vi "VIP_Post-Install Custom Action 2021.vi"(10 "Variant":variant) -> (0 "error out":errorcluster)   [LabVIEW 2021]
uses:
  <vilib>/Utility/sysdir.llb/System Directory Type.ctl
  <userlib>/_OpenG.lib/file/file.llb/Build Path - Traditional__ogtk.vi
  <userlib>/_OpenG.lib/lvzip/fileutil.llb/subVIs/FILE Rename (Path)__ogtk.vi
  <userlib>/_OpenG.lib/file/file.llb/File Exists - Scalar__ogtk.vi
  <resource>/dialog/lvconfig.llb/LV Config Read String.vi
  <resource>/dialog/lvconfig.llb/LV Config Write String.vi
  <vilib>/regexp/Match Regular Expression.xnode
  <userlib>/_OpenG.lib/file/file.llb/openg_file.lvlib
panel:
  # "POST INSTALL"
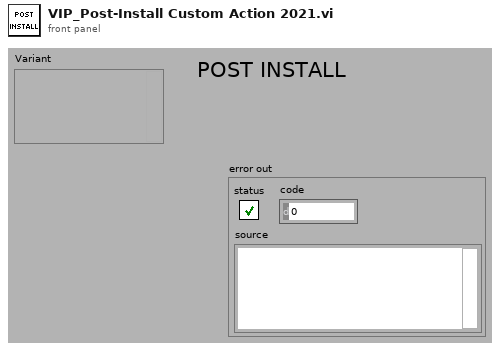
[diagram p1: front panel]
types:
  T1 = enum16{"open", "replace", "create", "open or create", "replace or create", "replace or create with confirmation"}
  T2 = typedef "System Directory Type.ctl" = i32
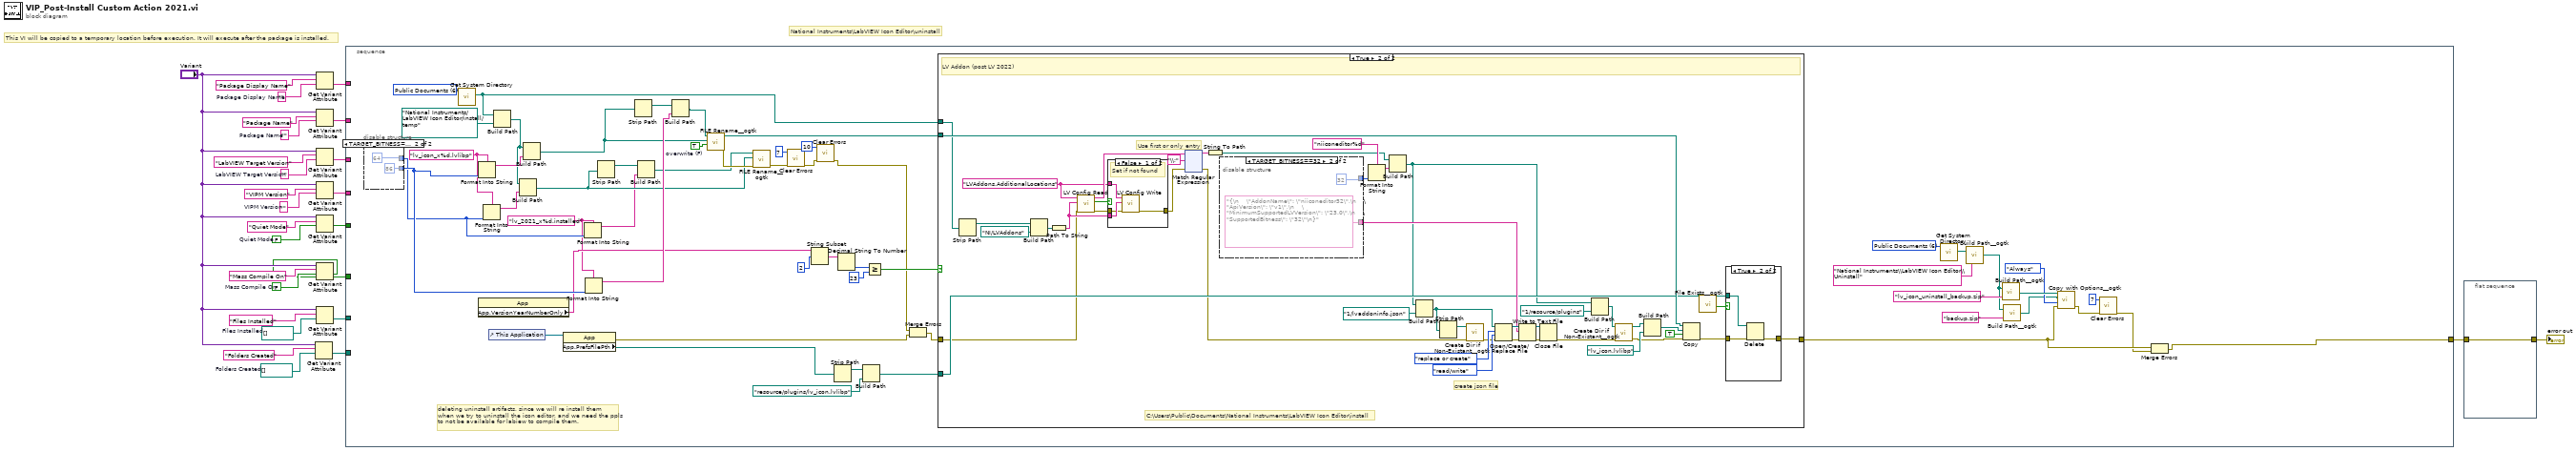
[diagram p0: block diagram]
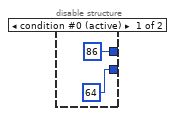
[diagram p2: hidden frame]
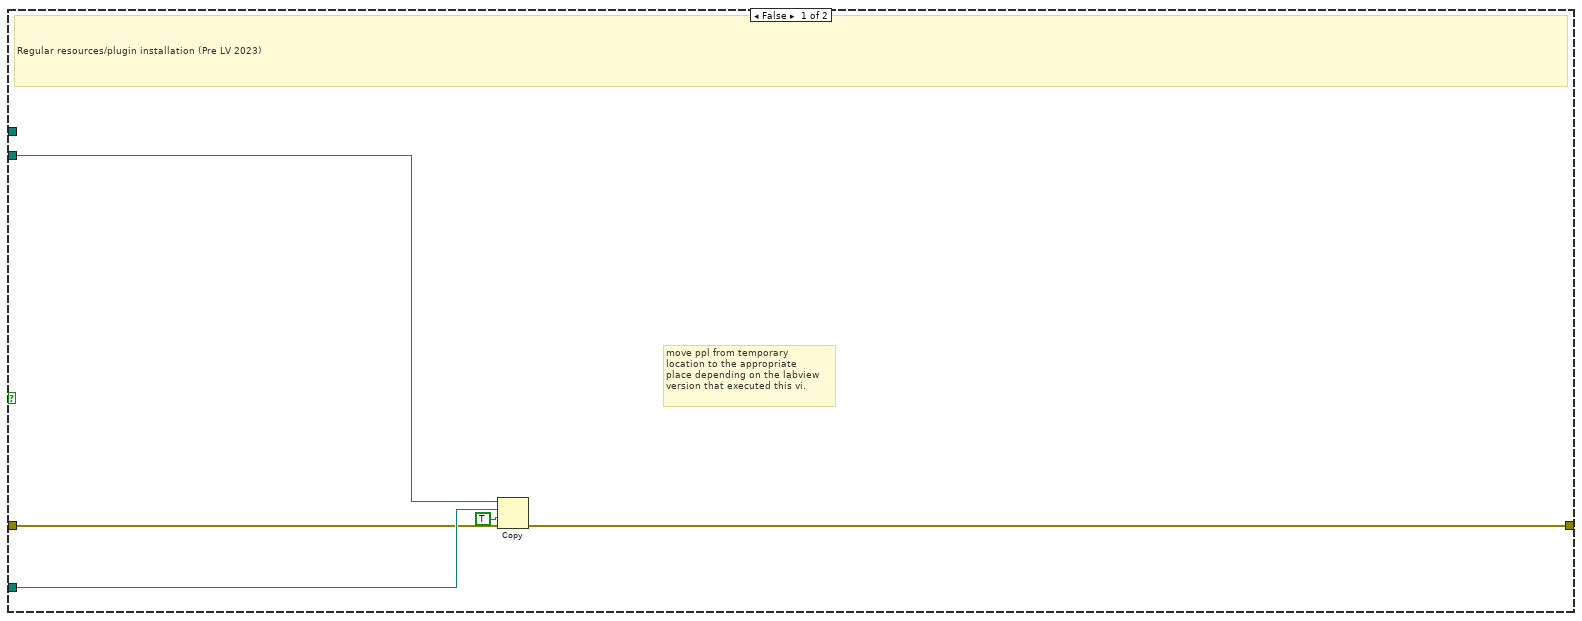
[diagram p3: hidden frame]
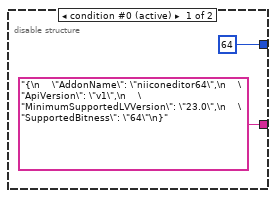
[diagram p6: hidden frame]
diagram:
  w11 = path[] []  # Folders Created
  w12 = path[] []  # Files Installed
  w16 = FALSE  # Mass Compile On
  w17 = ""  # Package Display Name
  w18 = FALSE  # Quiet Mode
  w21 = ""  # VIPM Version
  w23 = ""  # LabVIEW Target Version
  w25 = ""  # Package Name
  # "National Instruments\\LabVIEW Icon Editor\\uninstall"
  # "This VI will be copied to a temporary location before execution. It will execute after the package is installed."
  n1 = Get Variant Attribute(Variant="Variant", name="Folders Created", default value (empty Variant)=w11) -> (value=w3:path[])  [unwired: 1 in, 3 out]
  n2 = Get Variant Attribute(Variant="Variant", name="Package Display Name", default value (empty Variant)=w17) -> (value=w10:string)  [unwired: 1 in, 3 out]
  n3 = Get Variant Attribute(Variant="Variant", name="Package Name", default value (empty Variant)=w25) -> (value=w9:string)  [unwired: 1 in, 3 out]
  n4 = Get Variant Attribute(Variant="Variant", name="LabVIEW Target Version", default value (empty Variant)=w23) -> (value=w8:string)  [unwired: 1 in, 3 out]
  n5 = Get Variant Attribute(Variant="Variant", name="VIPM Version", default value (empty Variant)=w21) -> (value=w7:string)  [unwired: 1 in, 3 out]
  n6 = Get Variant Attribute(Variant="Variant", name="Quiet Mode", default value (empty Variant)=w18) -> (value=w6:bool)  [unwired: 1 in, 3 out]
  n7 = Get Variant Attribute(Variant="Variant", name="Mass Compile On", default value (empty Variant)=w16) -> (value=w5:bool)  [unwired: 1 in, 3 out]
  n8 = Get Variant Attribute(Variant="Variant", name="Files Installed", default value (empty Variant)=w12) -> (value=w4:path[])  [unwired: 1 in, 3 out]
  n9 = stacked-sequence {
    tunnel: [w28] -> w2
    tunnel: w10 -> [_]
    tunnel: w9 -> [_]
    tunnel: w8 -> [_]
    tunnel: w7 -> [_]
    tunnel: w6 -> [_]
    tunnel: w5 -> [_]
    tunnel: w4 -> [_]
    tunnel: w3 -> [_]
    frame #0 {
      w39 = "lv_2021_x%d.installed" ("format string")
      w58 = TRUE  # overwrite (F)
      w38 = "lv_icon_x%d.lvlibp" ("format string")
      w68 = T2 6 items=["User Home"=0, "User Desktop"=1, "User Documents"=2, "User Application Data"=3, "User Preferences"=4, "User Temporary"=5, "Public Documents"=6, "Public Application Data"=7, "Public Preferences"=8, "Public Cache"=13, "System Core Libraries"=9, "System Installed Libraries"=10, "Application Files"=11, "Boot Volume Root"=12] ("system directory type")
      w80 = T2 6 items=["User Home"=0, "User Desktop"=1, "User Documents"=2, "User Application Data"=3, "User Preferences"=4, "User Temporary"=5, "Public Documents"=6, "Public Application Data"=7, "Public Preferences"=8, "Public Cache"=13, "System Core Libraries"=9, "System Installed Libraries"=10, "Application Files"=11, "Boot Volume Root"=12] ("system directory type")
      # "deleting uninstall artifacts, since we will re install them\nwhen we try to uninstall the icon editor, and we need the ppls\nto not be available for labiew to compile them."
      n10 = disable-structure shown="TARGET_BITNESS==32" {
        disable-tunnel: [64 ("code") 86 ("code")] -> w57
        disable-tunnel: [86 ("code") 64 ("code")] -> w44
        frame condition #0 (active) {
        }
        frame condition #1 {
        }
      }
      n11 = call <vilib>:"Get System Directory.vi"("system directory type"=w80) -> ("system directory"=w29:path)  [unwired: 10 in]
      n12 = Format Into String(format string=w38, w57) -> (resulting string=w55:string)  [unwired: 2 in, 1 out]
      n13 = property class="App"() -> ("App.VersionYearNumberOnly"=w45:string)  [unwired: 2 in, 2 out]
      n14 = Format Into String(format string=w38, w44) -> (resulting string=w49:string)  [unwired: 2 in, 1 out]
      n15 = control-ref of="This Application"() -> (w79:refnum<vi>)
      n16 = Build Path(base path=w29, name or relative path=path "National Instruments/LabVIEW Icon Editor/install/temp" ("source path")) -> (appended path=w50:path)
      n17 = Build Path(base path=w50, name or relative path=w49) -> (appended path=w46:path)
      n18 = Build Path(base path=w50, name or relative path=w55) -> (appended path=w30:path)
      n19 = property class="App"(reference=w79) -> (error out=w59:errorcluster, "App.PrefsFilePth"=w63:path)  [unwired: 1 in, 1 out]
      n20 = Format Into String(format string=w39, w44) -> (resulting string=w43:string)  [unwired: 2 in, 1 out]
      n21 = Format Into String(format string=w39, w57) -> (resulting string=w52:string)  [unwired: 2 in, 1 out]
      n22 = Strip Path(path=w46) -> (stripped path=w47:path)  [unwired: 1 out]
      n23 = Strip Path(path=w30) -> (stripped path=w53:path)  [unwired: 1 out]
      n24 = Build Path(base path=w47, name or relative path=w43) -> (appended path=w42:path)
      n25 = Build Path(base path=w53, name or relative path=w52) -> (appended path=w51:path)
      n26 = call-poly <userlib>:"FILE Rename__ogtk.vi"("overwrite (F)"=w58, "source path"=w30, "target path"=w51) -> ("error out"=w48:errorcluster, "dup target path"=w54:path)  [unwired: 7 in]
      n27 = call-poly <userlib>:"FILE Rename__ogtk.vi"("error in (no error)"=w48, "source path"=w46, "target path"=w42) -> ("error out"=w41:errorcluster)  [unwired: 7 in, 1 out]
      n28 = call <vilib>:"Clear Errors.vi"("error in (no error)"=w41, "specific error code to clear (0: all)"=7) -> ("error out"=w37:errorcluster)  [unwired: 4 in, 1 out]
      n29 = String Subset(string=w45, offset (0)=2) -> (substring=w75:string)  [unwired: 1 in]
      n30 = call <vilib>:"Clear Errors.vi"("error in (no error)"=w37, "specific error code to clear (0: all)"=10) -> ("error out"=w36:errorcluster)  [unwired: 4 in, 1 out]
      n31 = Strip Path(path=w63) -> (stripped path=w65:path)  [unwired: 1 out]
      n32 = Decimal String To Number(string=w75) -> (number=w76:i32)  [unwired: 2 in, 1 out]
      n33 = Build Path(base path=w65, name or relative path=path "resource/plugins/lv_icon.lvlibp") -> (appended path=w62:path)
      n34 = Greater Or Equal?(x=w76, y=23) -> (x >= y?=w77:bool)
      n35 = Merge Errors(w36, w59) -> (w61:errorcluster)
      n36 = case shown="True" w77 {
        tunnel: w54 -> [w85 w112]
        tunnel: w61 -> [w86 w93]
        tunnel: w62 -> [w89 w110]
        tunnel: [w87 w116] -> w32
        tunnel: w29 -> [_ w97]
        frame False {
          # "move ppl from temporary\nlocation to the appropriate\nplace depending on the labview\nversion that executed this vi."
          # "Regular resources/plugin installation (Pre LV 2023)"
          n37 = Copy(8:w86, 9:TRUE ("overwrite (F)"), 10:w89, 11:w85) -> (0:w87:errorcluster)  [unwired: 1 in, 2 out]
        }
        frame True {
          w100 = "LVAddons.AdditionalLocations" ("key")
          # "Use first or only entry"
          # "C:\\Users\\Public\\Documents\\National Instruments\\LabVIEW Icon Editor\\install"
          # "create json file"
          # "LV Addon (post LV 2022)"
          n38 = Strip Path(path=w97) -> (stripped path=w101:path)  [unwired: 1 out]
          n39 = Build Path(base path=w101, name or relative path=path "NI/LVAddons") -> (appended path=w102:path)
          n40 = Path To String(path=w102) -> (string=w106:string)
          n41 = call-poly <resource>:"LV Config Read.vi"("error in"=w93, "default value"=w106, "key"=w100) -> ("error out"=w107:errorcluster, "found?"=w105:bool, "value"=w103:string)  [unwired: 2 in]
          n42 = case shown="False" w105 {
            tunnel: w100 -> [w136 _]
            tunnel: w106 -> [w135 _]
            tunnel: w107 -> [w134 w137]
            tunnel: [w133 w137] -> w108
            frame False {
              # "Set if not found"
              n43 = call-poly <resource>:"LV Config Write.vi"("error in (no error)"=w134, "value"=w135, "key"=w136) -> ("error out"=w133:errorcluster)  [unwired: 4 in]
            }
            frame True {
            }
          }
          n44 = xnode "Match Regular Expression"("input string"=w103, "regular expression"="\\;", "error in"=w108) -> ("before match"=w104:string, "error out"=w92:errorcluster)  [unwired: 3 in, 3 out]
          n45 = String To Path(string=w104) -> (path=w96:path)
          n46 = disable-structure shown="TARGET_BITNESS==32" {
            disable-tunnel: ["{\n    \"AddonName\": \"niiconeditor64\",\n    \"ApiVersion\": \"v1\",\n    \"MinimumSupportedLVVersion\": \"23.0\",\n    \"SupportedBitness\": \"64\"\n}" ("Tag Name") "{\n    \"AddonName\": \"niiconeditor32\",\n    \"ApiVersion\": \"v1\",\n    \"MinimumSupportedLVVersion\": \"23.0\",\n    \"SupportedBitness\": \"32\"\n}" ("Tag Name")] -> w126
            disable-tunnel: [64 ("code") 32 ("code")] -> w91
            frame condition #0 (active) {
            }
            frame condition #1 {
            }
          }
          n47 = Format Into String(format string="niiconeditor%d", w91) -> (resulting string=w125:string)  [unwired: 2 in, 1 out]
          n48 = Build Path(base path=w96, name or relative path=w125) -> (appended path=w90:path)
          n49 = Build Path(base path=w90, name or relative path=path "1/lvaddoninfo.json" ("Destination[i] Paths (Absolute)")) -> (appended path=w94:path)
          n50 = Strip Path(path=w94) -> (stripped path=w121:path)  [unwired: 1 out]
          n51 = call <userlib>:"Create Dir if Non-Existant__ogtk.vi"("error in (no error)"=w92, "Directory Path"=w121) -> ("error out"=w120:errorcluster)  [unwired: 7 in, 2 out]
          n52 = Open/Create/Replace File(file path (use dialog)=w94, error in=w120, operation (0:open)=T1."replace or create", access (0:read/write)=enum16{"read/write", "read-only", "write-only"}."read/write") -> (refnum out=w130:refnum<file>, error out=w131:errorcluster)  [unwired: 2 in, 1 out]
          n53 = Write to Text File(file (use dialog)=w130, text=w126, error in=w131) -> (refnum out=w129:refnum<file>, error out=w132:errorcluster)  [unwired: 1 in, 1 out]
          n54 = Close File(refnum=w129, error in=w132) -> (error out=w117:errorcluster)  [unwired: 1 out]
          n55 = Build Path(base path=w90, name or relative path=path "1/resource/plugins") -> (appended path=w119:path)
          n56 = call <userlib>:"Create Dir if Non-Existant__ogtk.vi"("error in (no error)"=w117, "Directory Path"=w119) -> ("error out"=w114:errorcluster, "dup Directory Path"=w118:path)  [unwired: 7 in, 1 out]
          n57 = Build Path(base path=w118, name or relative path=path "lv_icon.lvlibp" ("source path")) -> (appended path=w111:path)
          n58 = Copy(8:w114, 9:TRUE ("overwrite (F)"), 10:w111, 11:w112) -> (0:w109:errorcluster)  [unwired: 1 in, 2 out]
          n59 = call-poly <userlib>:"File Exists__ogtk.vi"("file path"=w110) -> ("exists"=w115:bool)  [unwired: 6 in, 1 out]
          n60 = case shown="True" w115 {
            tunnel: w109 -> [w255 w258]
            tunnel: w110 -> [_ w257]
            tunnel: [w255 w256] -> w116
            frame False {
            }
            frame True {
              n61 = Delete(path (use dialog)=w257, error in=w258) -> (error out=w256:errorcluster)  [unwired: 3 in, 2 out]
            }
          }
        }
      }
      n62 = call <vilib>:"Get System Directory.vi"("system directory type"=w68) -> ("system directory"=w72:path)  [unwired: 10 in]
      n63 = call-poly <userlib>:"Build Path__ogtk.vi"("name or relative path"="National Instruments\\LabVIEW Icon Editor\\Uninstall", "base path"=w72) -> ("appended path"=w60:path)
      n64 = call-poly <userlib>:"Build Path__ogtk.vi"("name or relative path"="lv_icon_uninstall_backup.zip", "base path"=w60) -> ("appended path"=w73:path)
      n65 = call-poly <userlib>:"Build Path__ogtk.vi"("name or relative path"="backup.zip", "base path"=w60) -> ("appended path"=w66:path)
      n66 = call <userlib>:"Copy with Options__ogtk.vi"("error in (no error)"=w32, "Replace Mode (Never)"=enum16{"Never", "Always", "If Newer"}."Always", "target path"=w66, "source path"=w73) -> ("error out"=w34:errorcluster)  [unwired: 6 in, 1 out]
      n67 = call <vilib>:"Clear Errors.vi"("error in (no error)"=w34, "specific error code to clear (0: all)"=7) -> ("error out"=w31:errorcluster)  [unwired: 4 in, 1 out]
      n68 = Merge Errors(w32, w31) -> (w28:errorcluster)
    }
  }
  n69 = flat-sequence {
    tunnel: w2 -> [w263]
    tunnel: [w263] -> w1
    frame #0 {
    }
  }
  "error out" <- w1
